vi "main.vi"() -> ()   [LabVIEW 2023] (continued)
00000004    8        68\t00\t97\tCC\t00\t16\t39\t8B\r\n      2262  1FFFFFFF   00000004    8        00\t00\tFF\tFF\tFF\tFF\tFF\tFF\r\n      2252  1FFFFFFF   00000004    8        00\t20\tFF\tFF\tFF\tFF\tFF\tFF\r\n      2247  1FFFFFFF   00000004    8        00\t00\tFF\tFF\tFF\tFF\tFF\tFF\r\n      2302  1FFFFFFF   00000004    8        00\t00\tFF\tFF\tFF\tFF\tFF\tFF\r\n      2293  18F106A7   00000004    8        00\tF7\tFF\tFF\tFF\tFF\tFF\t9E\r\n      2292  1FFFFFFF   00000004    8        00\t20\tFF\tFF\tFF\tFF\tFF\tFF\r\n      2283  0CF102A7   00000004    8        30\t75\tE0\t2E\t80\tFF\tFF\tFD\r\n      2283  0CF101A7   00000004    8        68\t00\t97\tCC\t00\t16\t39\t8C\r\n      2282  1FFFFFFF   00000004    8        00\t20\tFF\tFF\tFF\tFF\tFF\tFF\r\n      2272  1FFFFFFF   00000004    8        00\t20\tFF\tFF\tFF\tFF\tFF\tFF\r\n      2263  0CF102A7   00000004    8        30\t75\tE0\t2E\t80\tFF\tFF\tFD\r\n      2263  0CF101A7   00000004    8        68\t00\t97\tCC\t00\t16\t39\t8B\r\n      2262  1FFFFFFF   00000004    8        00\t00\tFF\tFF\tFF\tFF\tFF\tFF\r\n      2252  1FFFFFFF   00000004    8        00\t20\tFF\tFF\tFF\tFF\tFF\tFF\r\n      2303  0CF101A7   00000004    8        68\t00\t97\tCC\t00\t16\t39\t8D\r\n      2302  1FFFFFFF   00000004    8        00\t00\tFF\tFF\tFF\tFF\tFF\tFF\r\n      2293  18F106A7   00000004    8        00\tF7\tFF\tFF\tFF\tFF\tFF\t9E\r\n      2292  1FFFFFFF   00000004    8        00\t20\tFF\tFF\tFF\tFF\tFF\tFF\r\n      2283  0CF102A7   00000004    8        30\t75\tE0\t2E\t80\tFF\tFF\tFD\r\n      2283  0CF101A7   00000004    8        68\t00\t97\tCC\t00\t16\t39\t8C\r\n      2282  1FFFFFFF   00000004    8        00\t20\tFF\tFF\tFF\tFF\tFF\tFF\r\n      2272  1FFFFFFF   00000004    8        00\t20\tFF\tFF\tFF\tFF\tFF\tFF\r\n      2263  0CF102A7   00000004    8        30\t75\tE0\t2E\t80\tFF\tFF\tFD\r\n      2263  0CF101A7   00000004    8        68\t00\t97\tCC\t00\t16\t39\t8B\r\n      2262  1FFFFFFF   00000004    8        00\t00\tFF\tFF\tFF\tFF\tFF\tFF\r\n      2303  0CF102A7   00000004    8        30\t75\tE0\t2E\t80\tFF\tFF\tFD\r\n      2303  0CF101A7   00000004    8        68\t00\t97\tCC\t00\t16\t39\t8D\r\n      2302  1FFFFFFF   00000004    8        00\t00\tFF\tFF\tFF\tFF\tFF\tFF\r\n      2293  18F106A7   00000004    8        00\tF7\tFF\tFF\tFF\tFF\tFF\t9E\r\n      2292  1FFFFFFF   00000004    8        00\t20\tFF\tFF\tFF\tFF\tFF\tFF\r\n      2283  0CF102A7   00000004    8        30\t75\tE0\t2E\t80\tFF\tFF\tFD\r\n      2283  0CF101A7   00000004    8        68\t00\t97\tCC\t00\t16\t39\t8C\r\n      2282  1FFFFFFF   00000004    8        00\t20\tFF\tFF\tFF\tFF\tFF\tFF\r\n      2272  1FFFFFFF   00000004    8        00\t20\tFF\tFF\tFF\tFF\tFF\tFF\r\n      2263  0CF102A7   00000004    8        30\t75\tE0\t2E\t80\tFF\tFF\tFD\r\n      2263  0CF101A7   00000004    8        68\t00\t97\tCC\t00\t16\t39\t8B\r\n      2312  1FFFFFFF   00000004    8        00\t20\tFF\tFF\tFF\tFF\tFF\tFF\r\n      2303  0CF102A7   00000004    8        30\t75\tE0\t2E\t80\tFF\tFF\tFD\r\n      2303  0CF101A7   00000004    8        68\t00\t97\tCC\t00\t16\t39\t8D\r\n      2302  1FFFFFFF   00000004    8        00\t00\tFF\tFF\tFF\tFF\tFF\tFF\r\n      2293  18F106A7   00000004    8        00\tF7\tFF\tFF\tFF\tFF\tFF\t9E\r\n      2292  1FFFFFFF   00000004    8        00\t20\tFF\tFF\tFF\tFF\tFF\tFF\r\n      2283  0CF102A7   00000004    8        30\t75\tE0\t2E\t80\tFF\tFF\tFD\r\n      2283  0CF101A7   00000004    8        68\t00\t97\tCC\t00\t16\t39\t8C\r\n      2282  1FFFFFFF   00000004    8        00\t20\tFF\tFF\tFF\tFF\tFF\tFF\r\n      2272  1FFFFFFF   00000004    8        00\t20\tFF\tFF\tFF\tFF\tFF\tFF\r\n      2263  0CF102A7   00000004    8        30\t75\tE0\t2E\t80\tFF\tFF\tFD\r\n      2322  1FFFFFFF   00000004    8        00\t00\tFF\tFF\tFF\tFF\tFF\tFF\r\n      2312  1FFFFFFF   00000004    8        00\t20\tFF\tFF\tFF\tFF\tFF\tFF\r\n      2303  0CF102A7   00000004    8        30\t75\tE0\t2E\t80\tFF\tFF\tFD\r\n      2303  0CF101A7   00000004    8        68\t00\t97\tCC\t00\t16\t39\t8D\r\n      2302  1FFFFFFF   00000004    8        00\t00\tFF\tFF\tFF\tFF\tFF\tFF\r\n      2293  18F106A7   00000004    8        00\tF7\tFF\tFF\tFF\tFF\tFF\t9E\r\n      2292  1FFFFFFF   00000004    8        00\t20\tFF\tFF\tFF\tFF\tFF\tFF\r\n      2283  0CF102A7   00000004    8        30\t75\tE0\t2E\t80\tFF\tFF\tFD\r\n      2283  0CF101A7   00000004    8        68\t00\t97\tCC\t00\t16\t39\t8C\r\n      2282  1FFFFFFF   00000004    8        00\t20\tFF\tFF\tFF\tFF\tFF\tFF\r\n      2272  1FFFFFFF   00000004    8        00\t20\tFF\tFF\tFF\tFF\tFF\tFF\r\n      2323  0CF101A7   00000004    8        68\t00\t97\tCC\t00\t16\t39\t8E\r\n      2322  1FFFFFFF   00000004    8        00\t00\tFF\tFF\tFF\tFF\tFF\tFF\r\n      2312  1FFFFFFF   00000004    8        00\t20\tFF\tFF\tFF\tFF\tFF\tFF\r\n      2303  0CF102A7   00000004    8        30\t75\tE0\t2E\t80\tFF\tFF\tFD\r\n      2303  0CF101A7   00000004    8        68\t00\t97\tCC\t00\t16\t39\t8D\r\n      2302  1FFFFFFF   00000004    8        00\t00\tFF\tFF\tFF\tFF\tFF\tFF\r\n      2293  18F106A7   00000004    8        00\tF7\tFF\tFF\tFF\tFF\tFF\t9E\r\n      2292  1FFFFFFF   00000004    8        00\t20\tFF\tFF\tFF\tFF\tFF\tFF\r\n      2283  0CF102A7   00000004    8        30\t75\tE0\t2E\t80\tFF\tFF\tFD\r\n      2283  0CF101A7   00000004    8        68\t00\t97\tCC\t00\t16\t39\t8C\r\n      2282  1FFFFFFF   00000004    8        00\t20\tFF\tFF\tFF\tFF\tFF\tFF\r\n      2323  0CF102A7   00000004    8        30\t75\tE0\t2E\t80\tFF\tFF\tFD\r\n      2323  0CF101A7   00000004    8        68\t00\t97\tCC\t00\t16\t39\t8E\r\n      2322  1FFFFFFF   00000004    8        00\t00\tFF\tFF\tFF\tFF\tFF\tFF\r\n      2312  1FFFFFFF   00000004    8        00\t20\tFF\tFF\tFF\tFF\tFF\tFF\r\n      2303  0CF102A7   00000004    8        30\t75\tE0\t2E\t80\tFF\tFF\tFD\r\n      2303  0CF101A7   00000004    8        68\t00\t97\tCC\t00\t16\t39\t8D\r\n      2302  1FFFFFFF   00000004    8        00\t00\tFF\tFF\tFF\tFF\tFF\tFF\r\n      2293  18F106A7   00000004    8        00\tF7\tFF\tFF\tFF\tFF\tFF\t9E\r\n      2292  1FFFFFFF   00000004    8        00\t20\tFF\tFF\tFF\tFF\tFF\tFF\r\n      2283  0CF102A7   00000004    8        30\t75\tE0\t2E\t80\tFF\tFF\tFD\r\n      2283  0CF101A7   00000004    8        68\t00\t97\tCC\t00\t16\t39\t8C\r\n      2332  1FFFFFFF   00000004    8        00\t20\tFF\tFF\tFF\tFF\tFF\tFF\r\n      2323  0CF102A7   00000004    8        30\t75\tE0\t2E\t80\tFF\tFF\tFD\r\n      2323  0CF101A7   00000004    8        68\t00\t97\tCC\t00\t16\t39\t8E\r\n      2322  1FFFFFFF   00000004    8        00\t00\tFF\tFF\tFF\tFF\tFF\tFF\r\n      2312  1FFFFFFF   00000004    8        00\t20\tFF\tFF\tFF\tFF\tFF\tFF\r\n      2303  0CF102A7   00000004    8        30\t75\tE0\t2E\t80\tFF\tFF\tFD\r\n      2303  0CF101A7   00000004    8        68\t00\t97\tCC\t00\t16\t39\t8D\r\n      2302  1FFFFFFF   00000004    8        00\t00\tFF\tFF\tFF\tFF\tFF\tFF\r\n      2293  18F106A7   00000004    8        00\tF7\tFF\tFF\tFF\tFF\tFF\t9E\r\n      2292  1FFFFFFF   00000004    8        00\t20\tFF\tFF\tFF\tFF\tFF\tFF\r\n      2283  0CF102A7   00000004    8        30\t75\tE0\t2E\t80\tFF\tFF\tFD\r\n      2341  18F11FF0   00000004    8        FF\t3F\t90\t68\t88\t1B\t10\tFC\r\n      2332  1FFFFFFF   00000004    8        00\t20\tFF\tFF\tFF\tFF\tFF\tFF\r\n      2323  0CF102A7   00000004    8        30\t75\tE0\t2E\t80\tFF\tFF\tFD\r\n      2323  0CF101A7   00000004    8        68\t00\t97\tCC\t00\t16\t39\t8E\r\n      2322  1FFFFFFF   00000004    8        00\t00\tFF\tFF\tFF\tFF\tFF\tFF\r\n      2312  1FFFFFFF   00000004    8        00\t20\tFF\tFF\tFF\tFF\tFF\tFF\r\n      2303  0CF102A7   00000004    8        30\t75\tE0\t2E\t80\tFF\tFF\tFD\r\n      2303  0CF101A7   00000004    8        68\t00\t97\tCC\t00\t16\t39\t8D\r\n      2302  1FFFFFFF   00000004    8        00\t00\tFF\tFF\tFF\tFF\tFF\tFF\r\n      2293  18F106A7   00000004    8        00\tF7\tFF\tFF\tFF\tFF\tFF\t9E\r\n      2292  1FFFFFFF   00000004    8        00\t20\tFF\tFF\tFF\tFF\tFF\tFF\r\n      2342  18F120F0   00000004    8        2B\t75\t60\tB1\tB0\t01\tFF\tFF\r\n      2341  18F11FF0   00000004    8        FF\t3F\t90\t68\t88\t1B\t10\tFC\r\n      2332  1FFFFFFF   00000004    8        00\t20\tFF\tFF\tFF\tFF\tFF\tFF\r\n      2323  0CF102A7   00000004    8        30\t75\tE0\t2E\t80\tFF\tFF\tFD\r\n      2323  0CF101A7   00000004    8        68\t00\t97\tCC\t00\t16\t39\t8E\r\n      2322  1FFFFFFF   00000004    8        00\t00\tFF\tFF\tFF\tFF\tFF\tFF\r\n      2312  1FFFFFFF   00000004    8        00\t20\tFF\tFF\tFF\tFF\tFF\tFF\r\n      2303  0CF102A7   00000004    8        30\t75\tE0\t2E\t80\tFF\tFF\tFD\r\n      2303  0CF101A7   00000004    8        68\t00\t97\tCC\t00\t16\t39\t8D\r\n      2302  1FFFFFFF   00000004    8        00\t00\tFF\tFF\tFF\tFF\tFF\tFF\r\n      2293  18F106A7   00000004    8        00\tF7\tFF\tFF\tFF\tFF\tFF\t9E\r\n      2343  0CF101A7   00000004    8        68\t00\t97\tCC\t00\t16\t39\t8F\r\n      2342  18F120F0   00000004    8        2B\t75\t60\tB1\tB0\t01\tFF\tFF\r\n      2341  18F11FF0   00000004    8        FF\t3F\t90\t68\t88\t1B\t10\tFC\r\n      2332  1FFFFFFF   00000004    8        00\t20\tFF\tFF\tFF\tFF\tFF\tFF\r\n      2323  0CF102A7   00000004    8        30\t75\tE0\t2E\t80\tFF\tFF\tFD\r\n      2323  0CF101A7   00000004    8        68\t00\t97\tCC\t00\t16\t39\t8E\r\n      2322  1FFFFFFF   00000004    8        00\t00\tFF\tFF\tFF\tFF\tFF\tFF\r\n      2312  1FFFFFFF   00000004    8        00\t20\tFF\tFF\tFF\tFF\tFF\tFF\r\n      2303  0CF102A7   00000004    8        30\t75\tE0\t2E\t80\tFF\tFF\tFD\r\n      2303  0CF101A7   00000004    8        68\t00\t97\tCC\t00\t16\t39\t8D\r\n      2302  1FFFFFFF   00000004    8        00\t00\tFF\tFF\tFF\tFF\tFF\tFF\r\n      2343  0C3C4D4A   00000004    8        BE\tFF\tFF\t7F\t18\tFF\tFF\t4F\r\n      2343  0CF101A7   00000004    8        68\t00\t97\tCC\t00\t16\t39\t8F\r\n      2342  18F120F0   00000004    8        2B\t75\t60\tB1\tB0\t01\tFF\tFF\r\n      2341  18F11FF0   00000004    8        FF\t3F\t90\t68\t88\t1B\t10\tFC\r\n      2332  1FFFFFFF   00000004    8        00\t20\tFF\tFF\tFF\tFF\tFF\tFF\r\n      2323  0CF102A7   00000004    8        30\t75\tE0\t2E\t80\tFF\tFF\tFD\r\n      2323  0CF101A7   00000004    8        68\t00\t97\tCC\t00\t16\t39\t8E\r\n      2322  1FFFFFFF   00000004    8        00\t00\tFF\tFF\tFF\tFF\tFF\tFF\r\n      2312  1FFFFFFF   00000004    8        00\t20\tFF\tFF\tFF\tFF\tFF\tFF\r\n      2303  0CF102A7   00000004    8        30\t75\tE0\t2E\t80\tFF\tFF\tFD\r\n      2303  0CF101A7   00000004    8        68\t00\t97\tCC\t00\t16\t39\t8D\r\n      2344  0CF102A7   00000004    8        30\t75\tE0\t2E\t80\tFF\tFF\tFD\r\n      2343  0C3C4D4A   00000004    8        BE\tFF\tFF\t7F\t18\tFF\tFF\t4F\r\n      2343  0CF101A7   00000004    8        68\t00\t97\tCC\t00\t16\t39\t8F\r\n      2342  18F120F0   00000004    8        2B\t75\t60\tB1\tB0\t01\tFF\tFF\r\n      2341  18F11FF0   00000004    8        FF\t3F\t90\t68\t88\t1B\t10\tFC\r\n      2332  1FFFFFFF   00000004    8        00\t20\tFF\tFF\tFF\tFF\tFF\tFF\r\n      2323  0CF102A7   00000004    8        30\t75\tE0\t2E\t80\tFF\tFF\tFD\r\n      2323  0CF101A7   00000004    8        68\t00\t97\tCC\t00\t16\t39\t8E\r\n      2322  1FFFFFFF   00000004    8        00\t00\tFF\tFF\tFF\tFF\tFF\tFF\r\n      2312  1FFFFFFF   00000004    8        00\t20\tFF\tFF\tFF\tFF\tFF\tFF\r\n      2303  0CF102A7   00000004    8        30\t75\tE0\t2E\t80\tFF\tFF\tFD\r\n      2344  0CF103A7   00000004    8        17\t1F\t08\t60\tB1\t1F\t08\t4F\r\n      2344  0CF102A7   00000004    8        30\t75\tE0\t2E\t80\tFF\tFF\tFD\r\n      2343  0C3C4D4A   00000004    8        BE\tFF\tFF\t7F\t18\tFF\tFF\t4F\r\n      2343  0CF101A7   00000004    8        68\t00\t97\tCC\t00\t16\t39\t8F\r\n      2342  18F120F0   00000004    8        2B\t75\t60\tB1\tB0\t01\tFF\tFF\r\n      2341  18F11FF0   00000004    8        FF\t3F\t90\t68\t88\t1B\t10\tFC\r\n      2332  1FFFFFFF   00000004    8        00\t20\tFF\tFF\tFF\tFF\tFF\tFF\r\n      2323  0CF102A7   00000004    8        30\t75\tE0\t2E\t80\tFF\tFF\tFD\r\n      2323  0CF101A7   00000004    8        68\t00\t97\tCC\t00\t16\t39\t8E\r\n      2322  1FFFFFFF   00000004    8        00\t00\tFF\tFF\tFF\tFF\tFF\tFF\r\n      2312  1FFFFFFF   00000004    8        00\t20\tFF\tFF\tFF\tFF\tFF\tFF\r\n      2345  0CF104A7   00000004    8        F0\t60\t22\tFC\tFF\tFF\tFF\t4F\r\n      2344  0CF103A7   00000004    8        17\t1F\t08\t60\tB1\t1F\t08\t4F\r\n      2344  0CF102A7   00000004    8        30\t75\tE0\t2E\t80\tFF\tFF\tFD\r\n      2343  0C3C4D4A   00000004    8        BE\tFF\tFF\t7F\t18\tFF\tFF\t4F\r\n      2343  0CF101A7   00000004    8        68\t00\t97\tCC\t00\t16\t39\t8F\r\n      2342  18F120F0   00000004    8        2B\t75\t60\tB1\tB0\t01\tFF\tFF\r\n      2341  18F11FF0   00000004    8        FF\t3F\t90\t68\t88\t1B\t10\tFC\r\n      2332  1FFFFFFF   00000004    8        00\t20\tFF\tFF\tFF\tFF\tFF\tFF\r\n      2323  0CF102A7   00000004    8        30\t75\tE0\t2E\t80\tFF\tFF\tFD\r\n      2323  0CF101A7   00000004    8        68\t00\t97\tCC\t00\t16\t39\t8E\r\n      2322  1FFFFFFF   00000004    8        00\t00\tFF\tFF\tFF\tFF\tFF\tFF\r\n      2345  18F106A7   00000004    8        00\tF7\tFF\tFF\tFF\tFF\tFF\t9F\r\n      2345  0CF104A7   00000004    8        F0\t60\t22\tFC\tFF\tFF\tFF\t4F\r\n      2344  0CF103A7   00000004    8        17\t1F\t08\t60\tB1\t1F\t08\t4F\r\n      2344  0CF102A7   00000004    8        30\t75\tE0\t2E\t80\tFF\tFF\tFD\r\n      2343  0C3C4D4A   00000004    8        BE\tFF\tFF\t7F\t18\tFF\tFF\t4F\r\n      2343  0CF101A7   00000004    8        68\t00\t97\tCC\t00\t16\t39\t8F\r\n      2342  18F120F0   00000004    8        2B\t75\t60\tB1\tB0\t01\tFF\tFF\r\n      2341  18F11FF0   00000004    8        FF\t3F\t90\t68\t88\t1B\t10\tFC\r\n      2332  1FFFFFFF   00000004    8        00\t20\tFF\tFF\tFF\tFF\tFF\tFF\r\n      2323  0CF102A7   00000004    8        30\t75\tE0\t2E\t80\tFF\tFF\tFD\r\n      2323  0CF101A7   00000004    8        68\t00\t97\tCC\t00\t16\t39\t8E\r\n      2346  18F121F0   00000004    8        09\t19\t00\t00\tFF\tFF\tB0\t01\r\n      2345  18F106A7   00000004    8        00\tF7\tFF\tFF\tFF\tFF\tFF\t9F\r\n      2345  0CF104A7   00000004    8        F0\t60\t22\tFC\tFF\tFF\tFF\t4F\r\n      2344  0CF103A7   00000004    8        17\t1F\t08\t60\tB1\t1F\t08\t4F\r\n      2344  0CF102A7   00000004    8        30\t75\tE0\t2E\t80\tFF\tFF\tFD\r\n      2343  0C3C4D4A   00000004    8        BE\tFF\tFF\t7F\t18\tFF\tFF\t4F\r\n      2343  0CF101A7   00000004    8        68\t00\t97\tCC\t00\t16\t39\t8F\r\n      2342  18F120F0   00000004    8        2B\t75\t60\tB1\tB0\t01\tFF\tFF\r\n      2341  18F11FF0   00000004    8        FF\t3F\t90\t68\t88\t1B\t10\tFC\r\n      2332  1FFFFFFF   00000004    8        00\t20\tFF\tFF\tFF\tFF\tFF\tFF\r\n      2323  0CF102A7   00000004    8        30\t75\tE0\t2E\t80\tFF\tFF\tFD\r\n      2347  1FFFFFFF   00000004    8        00\t20\tFF\tFF\tFF\tFF\tFF\tFF\r\n      2346  18F121F0   00000004    8        09\t19\t00\t00\tFF\tFF\tB0\t01\r\n      2345  18F106A7   00000004    8        00\tF7\tFF\tFF\tFF\tFF\tFF\t9F\r\n      2345  0CF104A7   00000004    8        F0\t60\t22\tFC\tFF\tFF\tFF\t4F\r\n      2344  0CF103A7   00000004    8        17\t1F\t08\t60\tB1\t1F\t08\t4F\r\n      2344  0CF102A7   00000004    8        30\t75\tE0\t2E\t80\tFF\tFF\tFD\r\n      2343  0C3C4D4A   00000004    8        BE\tFF\tFF\t7F\t18\tFF\tFF\t4F\r\n      2343  0CF101A7   00000004    8        68\t00\t97\tCC\t00\t16\t39\t8F\r\n      2342  18F120F0   00000004    8        2B\t75\t60\tB1\tB0\t01\tFF\tFF\r\n      2341  18F11FF0   00000004    8        FF\t3F\t90\t68\t88\t1B\t10\tFC\r\n      2332  1FFFFFFF   00000004    8        00\t20\tFF\tFF\tFF\tFF\tFF\tFF\r\n      2352  1FFFFFFF   00000004    8        00\t20\tFF\tFF\tFF\tFF\tFF\tFF\r\n      2347  1FFFFFFF   00000004    8        00\t20\tFF\tFF\tFF\tFF\tFF\tFF\r\n      2346  18F121F0   00000004    8        09\t19\t00\t00\tFF\tFF\tB0\t01\r\n      2345  18F106A7   00000004    8        00\tF7\tFF\tFF\tFF\tFF\tFF\t9F\r\n      2345  0CF104A7   00000004    8        F0\t60\t22\tFC\tFF\tFF\tFF\t4F\r\n      2344  0CF103A7   00000004    8        17\t1F\t08\t60\tB1\t1F\t08\t4F\r\n      2344  0CF102A7   00000004    8        30\t75\tE0\t2E\t80\tFF\tFF\tFD\r\n      2343  0C3C4D4A   00000004    8        BE\tFF\tFF\t7F\t18\tFF\tFF\t4F\r\n      2343  0CF101A7   00000004    8        68\t00\t97\tCC\t00\t16\t39\t8F\r\n      2342  18F120F0   00000004    8        2B\t75\t60\tB1\tB0\t01\tFF\tFF\r\n      2341  18F11FF0   00000004    8        FF\t3F\t90\t68\t88\t1B\t10\tFC\r\n      2362  1FFFFFFF   00000004    8        00\t00\tFF\tFF\tFF\tFF\tFF\tFF\r\n      2352  1FFFFFFF   00000004    8        00\t20\tFF\tFF\tFF\tFF\tFF\tFF\r\n      2347  1FFFFFFF   00000004    8        00\t20\tFF\tFF\tFF\tFF\tFF\tFF\r\n      2346  18F121F0   00000004    8        09\t19\t00\t00\tFF\tFF\tB0\t01\r\n      2345  18F106A7   00000004    8        00\tF7\tFF\tFF\tFF\tFF\tFF\t9F\r\n      2345  0CF104A7   00000004    8        F0\t60\t22\tFC\tFF\tFF\tFF\t4F\r\n      2344  0CF103A7   00000004    8        17\t1F\t08\t60\tB1\t1F\t08\t4F\r\n      2344  0CF102A7   00000004    8        30\t75\tE0\t2E\t80\tFF\tFF\tFD\r\n      2343  0C3C4D4A   00000004    8        BE\tFF\tFF\t7F\t18\tFF\tFF\t4F\r\n      2343  0CF101A7   00000004    8        68\t00\t97\tCC\t00\t16\t39\t8F\r\n      2342  18F120F0   00000004    8        2B\t75\t60\tB1\tB0\t01\tFF\tFF\r\n      2363  0CF101A7   00000004    8        68\t00\t97\tCC\t00\t16\t39\t90\r\n      2362  1FFFFFFF   00000004    8        00\t00\tFF\tFF\tFF\tFF\tFF\tFF\r\n      2352  1FFFFFFF   00000004    8        00\t20\tFF\tFF\tFF\tFF\tFF\tFF\r\n      2347  1FFFFFFF   00000004    8        00\t20\tFF\tFF\tFF\tFF\tFF\tFF\r\n      2346  18F121F0   00000004    8        09\t19\t00\t00\tFF\tFF\tB0\t01\r\n      2345  18F106A7   00000004    8        00\tF7\tFF\tFF\tFF\tFF\tFF\t9F\r\n      2345  0CF104A7   00000004    8        F0\t60\t22\tFC\tFF\tFF\tFF\t4F\r\n      2344  0CF103A7   00000004    8        17\t1F\t08\t60\tB1\t1F\t08\t4F\r\n      2344  0CF102A7   00000004    8        30\t75\tE0\t2E\t80\tFF\tFF\tFD\r\n      2343  0C3C4D4A   00000004    8        BE\tFF\tFF\t7F\t18\tFF\tFF\t4F\r\n      2343  0CF101A7   00000004    8        68\t00\t97\tCC\t00\t16\t39\t8F\r\n      2363  0CF102A7   00000004    8        30\t75\tE0\t2E\t80\tFF\tFF\tFD\r\n      2363  0CF101A7   00000004    8        68\t00\t97\tCC\t00\t16\t39\t90\r\n      2362  1FFFFFFF   00000004    8        00\t00\tFF\tFF\tFF\tFF\tFF\tFF\r\n      2352  1FFFFFFF   00000004    8        00\t20\tFF\tFF\tFF\tFF\tFF\tFF\r\n      2347  1FFFFFFF   00000004    8        00\t20\tFF\tFF\tFF\tFF\tFF\tFF\r\n      2346  18F121F0   00000004    8        09\t19\t00\t00\tFF\tFF\tB0\t01\r\n      2345  18F106A7   00000004    8        00\tF7\tFF\tFF\tFF\tFF\tFF\t9F\r\n      2345  0CF104A7   00000004    8        F0\t60\t22\tFC\tFF\tFF\tFF\t4F\r\n      2344  0CF103A7   00000004    8        17\t1F\t08\t60\tB1\t1F\t08\t4F\r\n      2344  0CF102A7   00000004    8        30\t75\tE0\t2E\t80\tFF\tFF\tFD\r\n      2343  0C3C4D4A   00000004    8        BE\tFF\tFF\t7F\t18\tFF\tFF\t4F\r\n      2372  1FFFFFFF   00000004    8        00\t20\tFF\tFF\tFF\tFF\tFF\tFF\r\n      2363  0CF102A7   00000004    8        30\t75\tE0\t2E\t80\tFF\tFF\tFD\r\n      2363  0CF101A7   00000004    8        68\t00\t97\tCC\t00\t16\t39\t90\r\n      2362  1FFFFFFF   00000004    8        00\t00\tFF\tFF\tFF\tFF\tFF\tFF\r\n      2352  1FFFFFFF   00000004    8        00\t20\tFF\tFF\tFF\tFF\tFF\tFF\r\n      2347  1FFFFFFF   00000004    8        00\t20\tFF\tFF\tFF\tFF\tFF\tFF\r\n      2346  18F121F0   00000004    8        09\t19\t00\t00\tFF\tFF\tB0\t01\r\n      2345  18F106A7   00000004    8        00\tF7\tFF\tFF\tFF\tFF\tFF\t9F\r\n      2345  0CF104A7   00000004    8        F0\t60\t22\tFC\tFF\tFF\tFF\t4F\r\n      2344  0CF103A7   00000004    8        17\t1F\t08\t60\tB1\t1F\t08\t4F\r\n      2344  0CF102A7   00000004    8        30\t75\tE0\t2E\t80\tFF\tFF\tFD\r\n      2382  1FFFFFFF   00000004    8        00\t20\tFF\tFF\tFF\tFF\tFF\tFF\r\n      2372  1FFFFFFF   00000004    8        00\t20\tFF\tFF\tFF\tFF\tFF\tFF\r\n      2363  0CF102A7   00000004    8        30\t75\tE0\t2E\t80\tFF\tFF\tFD\r\n      2363  0CF101A7   00000004    8        68\t00\t97\tCC\t00\t16\t39\t90\r\n      2362  1FFFFFFF   00000004    8        00\t00\tFF\tFF\tFF\tFF\tFF\tFF\r\n      2352  1FFFFFFF   00000004    8        00\t20\tFF\tFF\tFF\tFF\tFF\tFF\r\n      2347  1FFFFFFF   00000004    8        00\t20\tFF\tFF\tFF\tFF\tFF\tFF\r\n      2346  18F121F0   00000004    8        09\t19\t00\t00\tFF\tFF\tB0\t01\r\n      2345  18F106A7   00000004    8        00\tF7\tFF\tFF\tFF\tFF\tFF\t9F\r\n      2345  0CF104A7   00000004    8        F0\t60\t22\tFC\tFF\tFF\tFF\t4F\r\n      2344  0CF103A7   00000004    8        17\t1F\t08\t60\tB1\t1F\t08\t4F\r\n      2383  0CF101A7   00000004    8        68\t00\t97\tCC\t00\t16\t39\t91\r\n      2382  1FFFFFFF   00000004    8        00\t20\tFF\tFF\tFF\tFF\tFF\tFF\r\n      2372  1FFFFFFF   00000004    8        00\t20\tFF\tFF\tFF\tFF\tFF\tFF\r\n      2363  0CF102A7   00000004    8        30\t75\tE0\t2E\t80\tFF\tFF\tFD\r\n      2363  0CF101A7   00000004    8        68\t00\t97\tCC\t00\t16\t39\t90\r\n      2362  1FFFFFFF   00000004    8        00\t00\tFF\tFF\tFF\tFF\tFF\tFF\r\n      2352  1FFFFFFF   00000004    8        00\t20\tFF\tFF\tFF\tFF\tFF\tFF\r\n      2347  1FFFFFFF   00000004    8        00\t20\tFF\tFF\tFF\tFF\tFF\tFF\r\n      2346  18F121F0   00000004    8        09\t19\t00\t00\tFF\tFF\tB0\t01\r\n      2345  18F106A7   00000004    8        00\tF7\tFF\tFF\tFF\tFF\tFF\t9F\r\n      2345  0CF104A7   00000004    8        F0\t60\t22\tFC\tFF\tFF\tFF\t4F\r\n      2383  0CF102A7   00000004    8        30\t75\tE0\t2E\t80\tFF\tFF\tFD\r\n      2383  0CF101A7   00000004    8        68\t00\t97\tCC\t00\t16\t39\t91\r\n      2382  1FFFFFFF   00000004    8        00\t20\tFF\tFF\tFF\tFF\tFF\tFF\r\n      2372  1FFFFFFF   00000004    8        00\t20\tFF\tFF\tFF\tFF\tFF\tFF\r\n      2363  0CF102A7   00000004    8        30\t75\tE0\t2E\t80\tFF\tFF\tFD\r\n      2363  0CF101A7   00000004    8        68\t00\t97\tCC\t00\t16\t39\t90\r\n      2362  1FFFFFFF   00000004    8        00\t00\tFF\tFF\tFF\tFF\tFF\tFF\r\n      2352  1FFFFFFF   00000004    8        00\t20\tFF\tFF\tFF\tFF\tFF\tFF\r\n      2347  1FFFFFFF   00000004    8        00\t20\tFF\tFF\tFF\tFF\tFF\tFF\r\n      2346  18F121F0   00000004    8        09\t19\t00\t00\tFF\tFF\tB0\t01\r\n      2345  18F106A7   00000004    8        00\tF7\tFF\tFF\tFF\tFF\tFF\t9F\r\n      2392  1FFFFFFF   00000004    8        00\t20\tFF\tFF\tFF\tFF\tFF\tFF\r\n      2383  0CF102A7   00000004    8        30\t75\tE0\t2E\t80\tFF\tFF\tFD\r\n      2383  0CF101A7   00000004    8        68\t00\t97\tCC\t00\t16\t39\t91\r\n      2382  1FFFFFFF   00000004    8        00\t20\tFF\tFF\tFF\tFF\tFF\tFF\r\n      2372  1FFFFFFF   00000004    8        00\t20\tFF\tFF\tFF\tFF\tFF\tFF\r\n      2363  0CF102A7   00000004    8        30\t75\tE0\t2E\t80\tFF\tFF\tFD\r\n      2363  0CF101A7   00000004    8        68\t00\t97\tCC\t00\t16\t39\t90\r\n      2362  1FFFFFFF   00000004    8        00\t00\tFF\tFF\tFF\tFF\tFF\tFF\r\n      2352  1FFFFFFF   00000004    8        00\t20\tFF\tFF\tFF\tFF\tFF\tFF\r\n      2347  1FFFFFFF   00000004    8        00\t20\tFF\tFF\tFF\tFF\tFF\tFF\r\n      2346  18F121F0   00000004    8        09\t19\t00\t00\tFF\tFF\tB0\t01\r\n      2393  18F106A7   00000004    8        00\tF7\tFF\tFF\tFF\tFF\tFF\tA0\r\n      2392  1FFFFFFF   00000004    8        00\t20\tFF\tFF\tFF\tFF\tFF\tFF\r\n      2383  0CF102A7   00000004    8        30\t75\tE0\t2E\t80\tFF\tFF\tFD\r\n      2383  0CF101A7   00000004    8        68\t00\t97\tCC\t00\t16\t39\t91\r\n      2382  1FFFFFFF   00000004    8        00\t20\tFF\tFF\tFF\tFF\tFF\tFF\r\n      2372  1FFFFFFF   00000004    8        00\t20\tFF\tFF\tFF\tFF\tFF\tFF\r\n      2363  0CF102A7   00000004    8        30\t75\tE0\t2E\t80\tFF\tFF\tFD\r\n      2363  0CF101A7   00000004    8        68\t00\t97\tCC\t00\t16\t39\t90\r\n      2362  1FFFFFFF   00000004    8        00\t00\tFF\tFF\tFF\tFF\tFF\tFF\r\n      2352  1FFFFFFF   00000004    8        00\t20\tFF\tFF\tFF\tFF\tFF\tFF\r\n      2347  1FFFFFFF   00000004    8        00\t20\tFF\tFF\tFF\tFF\tFF\tFF\r\n      2402  1FFFFFFF   00000004    8        00\t00\tFF\tFF\tFF\tFF\tFF\tFF\r\n      2393  18F106A7   00000004    8        00\tF7\tFF\tFF\tFF\tFF\tFF\tA0\r\n      2392  1FFFFFFF   00000004    8        00\t20\tFF\tFF\tFF\tFF\tFF\tFF\r\n      2383  0CF102A7   00000004    8        30\t75\tE0\t2E\t80\tFF\tFF\tFD\r\n      2383  0CF101A7   00000004    8        68\t00\t97\tCC\t00\t16\t39\t91\r\n      2382  1FFFFFFF   00000004    8        00\t20\tFF\tFF\tFF\tFF\tFF\tFF\r\n      2372  1FFFFFFF   00000004    8        00\t20\tFF\tFF\tFF\tFF\tFF\tFF\r\n      2363  0CF102A7   00000004    8        30\t75\tE0\t2E\t80\tFF\tFF\tFD\r\n      2363  0CF101A7   00000004    8        68\t00\t97\tCC\t00\t16\t39\t90\r\n      2362  1FFFFFFF   00000004    8        00\t00\tFF\tFF\tFF\tFF\tFF\tFF\r\n      2352  1FFFFFFF   00000004    8        00\t20\tFF\tFF\tFF\tFF\tFF\tFF\r\n      2403  0CF101A7   00000004    8        68\t00\t97\tCC\t00\t16\t39\t92\r\n      2402  1FFFFFFF   00000004    8        00\t00\tFF\tFF\tFF\tFF\tFF\tFF\r\n      2393  18F106A7   00000004    8        00\tF7\tFF\tFF\tFF\tFF\tFF\tA0\r\n      2392  1FFFFFFF   00000004    8        00\t20\tFF\tFF\tFF\tFF\tFF\tFF\r\n      2383  0CF102A7   00000004    8        30\t75\tE0\t2E\t80\tFF\tFF\tFD\r\n      2383  0CF101A7   00000004    8        68\t00\t97\tCC\t00\t16\t39\t91\r\n      2382  1FFFFFFF   00000004    8        00\t20\tFF\tFF\tFF\tFF\tFF\tFF\r\n      2372  1FFFFFFF   00000004    8        00\t20\tFF\tFF\tFF\tFF\tFF\tFF\r\n      2363  0CF102A7   00000004    8        30\t75\tE0\t2E\t80\tFF\tFF\tFD\r\n      2363  0CF101A7   00000004    8        68\t00\t97\tCC\t00\t16\t39\t90\r\n      2362  1FFFFFFF   00000004    8        00\t00\tFF\tFF\tFF\tFF\tFF\tFF\r\n      2403  0CF102A7   00000004    8        30\t75\tE0\t2E\t80\tFF\tFF\tFD\r\n      2403  0CF101A7   00000004    8        68\t00\t97\tCC\t00\t16\t39\t92\r\n      2402  1FFFFFFF   00000004    8        00\t00\tFF\tFF\tFF\tFF\tFF\tFF\r\n      2393  18F106A7   00000004    8        00\tF7\tFF\tFF\tFF\tFF\tFF\tA0\r\n      2392  1FFFFFFF   00000004    8        00\t20\tFF\tFF\tFF\tFF\tFF\tFF\r\n      2383  0CF102A7   00000004    8        30\t75\tE0\t2E\t80\tFF\tFF\tFD\r\n      2383  0CF101A7   00000004    8        68\t00\t97\tCC\t00\t16\t39\t91\r\n      2382  1FFFFFFF   00000004    8        00\t20\tFF\tFF\tFF\tFF\tFF\tFF\r\n      2372  1FFFFFFF   00000004    8        00\t20\tFF\tFF\tFF\tFF\tFF\tFF\r\n      2363  0CF102A7   00000004    8        30\t75\tE0\t2E\t80\tFF\tFF\tFD\r\n      2363  0CF101A7   00000004    8        68\t00\t97\tCC\t00\t16\t39\t90\r\n      2412  1FFFFFFF   00000004    8        00\t20\tFF\tFF\tFF\tFF\tFF\tFF\r\n      2403  0CF102A7   00000004    8        30\t75\tE0\t2E\t80\tFF\tFF\tFD\r\n      2403  0CF101A7   00000004    8        68\t00\t97\tCC\t00\t16\t39\t92\r\n      2402  1FFFFFFF   00000004    8        00\t00\tFF\tFF\tFF\tFF\tFF\tFF\r\n      2393  18F106A7   00000004    8        00\tF7\tFF\tFF\tFF\tFF\tFF\tA0\r\n      2392  1FFFFFFF   00000004    8        00\t20\tFF\tFF\tFF\tFF\tFF\tFF\r\n      2383  0CF102A7   00000004    8        30\t75\tE0\t2E\t80\tFF\tFF\tFD\r\n      2383  0CF101A7   00000004    8        68\t00\t97\tCC\t00\t16\t39\t91\r\n      2382  1FFFFFFF   00000004    8        00\t20\tFF\tFF\tFF\tFF\tFF\tFF\r\n      2372  1FFFFFFF   00000004    8        00\t20\tFF\tFF\tFF\tFF\tFF\tFF\r\n      2363  0CF102A7   00000004    8        30\t75\tE0\t2E\t80\tFF\tFF\tFD\r\n      2422  1FFFFFFF   00000004    8        00\t00\tFF\tFF\tFF\tFF\tFF\tFF\r\n      2412  1FFFFFFF   00000004    8        00\t20\tFF\tFF\tFF\tFF\tFF\tFF\r\n      2403  0CF102A7   00000004    8        30\t75\tE0\t2E\t80\tFF\tFF\tFD\r\n      2403  0CF101A7   00000004    8        68\t00\t97\tCC\t00\t16\t39\t92\r\n      2402  1FFFFFFF   00000004    8        00\t00\tFF\tFF\tFF\tFF\tFF\tFF\r\n      2393  18F106A7   00000004    8        00\tF7\tFF\tFF\tFF\tFF\tFF\tA0\r\n      2392  1FFFFFFF   00000004    8        00\t20\tFF\tFF\tFF\tFF\tFF\tFF\r\n      2383  0CF102A7   00000004    8        30\t75\tE0\t2E\t80\tFF\tFF\tFD\r\n      2383  0CF101A7   00000004    8        68\t00\t97\tCC\t00\t16\t39\t91\r\n      2382  1FFFFFFF   00000004    8        00\t20\tFF\tFF\tFF\tFF\tFF\tFF\r\n      2372  1FFFFFFF   00000004    8        00\t20\tFF\tFF\tFF\tFF\tFF\tFF\r\n      2423  0CF101A7   00000004    8        68\t00\t97\tCC\t00\t16\t39\t93\r\n      2422  1FFFFFFF   00000004    8        00\t00\tFF\tFF\tFF\tFF\tFF\tFF\r\n      2412  1FFFFFFF   00000004    8        00\t20\tFF\tFF\tFF\tFF\tFF\tFF\r\n      2403  0CF102A7   00000004    8        30\t75\tE0\t2E\t80\tFF\tFF\tFD\r\n      2403  0CF101A7   00000004    8        68\t00\t97\tCC\t00\t16\t39\t92\r\n      2402  1FFFFFFF   00000004    8        00\t00\tFF\tFF\tFF\tFF\tFF\tFF\r\n      2393  18F106A7   00000004    8        00\tF7\tFF\tFF\tFF\tFF\tFF\tA0\r\n      2392  1FFFFFFF   00000004    8        00\t20\tFF\tFF\tFF\tFF\tFF\tFF\r\n      2383  0CF102A7   00000004    8        30\t75\tE0\t2E\t80\tFF\tFF\tFD\r\n      2383  0CF101A7   00000004    8        68\t00\t97\tCC\t00\t16\t39\t91\r\n      2382  1FFFFFFF   00000004    8        00\t20\tFF\tFF\tFF\tFF\tFF\tFF\r\n      2423  0CF102A7   00000004    8        30\t75\tE0\t2E\t80\tFF\tFF\tFD\r\n      2423  0CF101A7   00000004    8        68\t00\t97\tCC\t00\t16\t39\t93\r\n      2422  1FFFFFFF   00000004    8        00\t00\tFF\tFF\tFF\tFF\tFF\tFF\r\n      2412  1FFFFFFF   00000004    8        00\t20\tFF\tFF\tFF\tFF\tFF\tFF\r\n      2403  0CF102A7   00000004    8        30\t75\tE0\t2E\t80\tFF\tFF\tFD\r\n      2403  0CF101A7   00000004    8        68\t00\t97\tCC\t00\t16\t39\t92\r\n      2402  1FFFFFFF   00000004    8        00\t00\tFF\tFF\tFF\tFF\tFF\tFF\r\n      2393  18F106A7   00000004    8        00\tF7\tFF\tFF\tFF\tFF\tFF\tA0\r\n      2392  1FFFFFFF   00000004    8        00\t20\tFF\tFF\tFF\tFF\tFF\tFF\r\n      2383  0CF102A7   00000004    8        30\t75\tE0\t2E\t80\tFF\tFF\tFD\r\n      2383  0CF101A7   00000004    8        68\t00\t97\tCC\t00\t16\t39\t91\r\n      2432  1FFFFFFF   00000004    8        00\t20\tFF\tFF\tFF\tFF\tFF\tFF\r\n      2423  0CF102A7   00000004    8        30\t75\tE0\t2E\t80\tFF\tFF\tFD\r\n      2423  0CF101A7   00000004    8        68\t00\t97\tCC\t00\t16\t39\t93\r\n      2422  1FFFFFFF   00000004    8        00\t00\tFF\tFF\tFF\tFF\tFF\tFF\r\n      2412  1FFFFFFF   00000004    8        00\t20\tFF\tFF\tFF\tFF\tFF\tFF\r\n      2403  0CF102A7   00000004    8        30\t75\tE0\t2E\t80\tFF\tFF\tFD\r\n      2403  0CF101A7   00000004    8        68\t00\t97\tCC\t00\t16\t39\t92\r\n      2402  1FFFFFFF   00000004    8        00\t00\tFF\tFF\tFF\tFF\tFF\tFF\r\n      2393  18F106A7   00000004    8        00\tF7\tFF\tFF\tFF\tFF\tFF\tA0\r\n      2392  1FFFFFFF   00000004    8        00\t20\tFF\tFF\tFF\tFF\tFF\tFF\r\n      2383  0CF102A7   00000004    8        30\t75\tE0\t2E\t80\tFF\tFF\tFD\r\n      2441  18F11FF0   00000004    8        FF\t3F\t90\t68\t88\t1B\t10\t0C\r\n      2432  1FFFFFFF   00000004    8        00\t20\tFF\tFF\tFF\tFF\tFF\tFF\r\n      2423  0CF102A7   00000004    8        30\t75\tE0\t2E\t80\tFF\tFF\tFD\r\n      2423  0CF101A7   00000004    8        68\t00\t97\tCC\t00\t16\t39\t93\r\n      2422  1FFFFFFF   00000004    8        00\t00\tFF\tFF\tFF\tFF\tFF\tFF\r\n      2412  1FFFFFFF   00000004    8        00\t20\tFF\tFF\tFF\tFF\tFF\tFF\r\n      2403  0CF102A7   00000004    8        30\t75\tE0\t2E\t80\tFF\tFF\tFD\r\n      2403  0CF101A7   00000004    8        68\t00\t97\tCC\t00\t16\t39\t92\r\n      2402  1FFFFFFF   00000004    8        00\t00\tFF\tFF\tFF\tFF\tFF\tFF\r\n      2393  18F106A7   00000004    8        00\tF7\tFF\tFF\tFF\tFF\tFF\tA0\r\n      2392  1FFFFFFF   00000004    8        00\t20\tFF\tFF\tFF\tFF\tFF\tFF\r\n      2442  18F120F0   00000004    8        2B\t75\t60\tB1\tB0\t01\tFF\tFF\r\n      2441  18F11FF0   00000004    8        FF\t3F\t90\t68\t88\t1B\t10\t0C\r\n      2432  1FFFFFFF   00000004    8        00\t20\tFF\tFF\tFF\tFF\tFF\tFF\r\n      2423  0CF102A7   00000004    8        30\t75\tE0\t2E\t80\tFF\tFF\tFD\r\n      2423  0CF101A7   00000004    8        68\t00\t97\tCC\t00\t16\t39\t93\r\n      2422  1FFFFFFF   00000004    8        00\t00\tFF\tFF\tFF\tFF\tFF\tFF\r\n      2412  1FFFFFFF   00000004    8        00\t20\tFF\tFF\tFF\tFF\tFF\tFF\r\n      2403  0CF102A7   00000004    8        30\t75\tE0\t2E\t80\tFF\tFF\tFD\r\n      2403  0CF101A7   00000004    8        68\t00\t97\tCC\t00\t16\t39\t92\r\n      2402  1FFFFFFF   00000004    8        00\t00\tFF\tFF\tFF\tFF\tFF\tFF\r\n      2393  18F106A7   00000004    8        00\tF7\tFF\tFF\tFF\tFF\tFF\tA0\r\n      2443  0CF101A7   00000004    8        68\t00\t97\tCC\t00\t16\t39\t94\r\n      2442  18F120F0   00000004    8        2B\t75\t60\tB1\tB0\t01\tFF\tFF\r\n      2441  18F11FF0   00000004    8        FF\t3F\t90\t68\t88\t1B\t10\t0C\r\n      2432  1FFFFFFF   00000004    8        00\t20\tFF\tFF\tFF\tFF\tFF\tFF\r\n      2423  0CF102A7   00000004    8        30\t75\tE0\t2E\t80\tFF\tFF\tFD\r\n      2423  0CF101A7   00000004    8        68\t00\t97\tCC\t00\t16\t39\t93\r\n      2422  1FFFFFFF   00000004    8        00\t00\tFF\tFF\tFF\tFF\tFF\tFF\r\n      2412  1FFFFFFF   00000004    8        00\t20\tFF\tFF\tFF\tFF\tFF\tFF\r\n      2403  0CF102A7   00000004    8        30\t75\tE0\t2E\t80\tFF\tFF\tFD\r\n      2403  0CF101A7   00000004    8        68\t00\t97\tCC\t00\t16\t39\t92\r\n      2402  1FFFFFFF   00000004    8        00\t00\tFF\tFF\tFF\tFF\tFF\tFF\r\n      2443  0C3C4D4A   00000004    8        BE\tFF\tFF\t7F\t18\tFF\tFF\t50\r\n      2443  0CF101A7   00000004    8        68\t00\t97\tCC\t00\t16\t39\t94\r\n      2442  18F120F0   00000004    8        2B\t75\t60\tB1\tB0\t01\tFF\tFF\r\n      2441  18F11FF0   00000004    8        FF\t3F\t90\t68\t88\t1B\t10\t0C\r\n      2432  1FFFFFFF   00000004    8        00\t20\tFF\tFF\tFF\tFF\tFF\tFF\r\n      2423  0CF102A7   00000004    8        30\t75\tE0\t2E\t80\tFF\tFF\tFD\r\n      2423  0CF101A7   00000004    8        68\t00\t97\tCC\t00\t16\t39\t93\r\n      2422  1FFFFFFF   00000004    8        00\t00\tFF\tFF\tFF\tFF\tFF\tFF\r\n      2412  1FFFFFFF   00000004    8        00\t20\tFF\tFF\tFF\tFF\tFF\tFF\r\n      2403  0CF102A7   00000004    8        30\t75\tE0\t2E\t80\tFF\tFF\tFD\r\n      2403  0CF101A7   00000004    8        68\t00\t97\tCC\t00\t16\t39\t92\r\n      2444  0CF102A7   00000004    8        30\t75\tE0\t2E\t80\tFF\tFF\tFD\r\n      2443  0C3C4D4A   00000004    8        BE\tFF\tFF\t7F\t18\tFF\tFF\t50\r\n      2443  0CF101A7   00000004    8        68\t00\t97\tCC\t00\t16\t39\t94\r\n      2442  18F120F0   00000004    8        2B\t75\t60\tB1\tB0\t01\tFF\tFF\r\n      2441  18F11FF0   00000004    8        FF\t3F\t90\t68\t88\t1B\t10\t0C\r\n      2432  1FFFFFFF   00000004    8        00\t20\tFF\tFF\tFF\tFF\tFF\tFF\r\n      2423  0CF102A7   00000004    8        30\t75\tE0\t2E\t80\tFF\tFF\tFD\r\n      2423  0CF101A7   00000004    8        68\t00\t97\tCC\t00\t16\t39\t93\r\n      2422  1FFFFFFF   00000004    8        00\t00\tFF\tFF\tFF\tFF\tFF\tFF\r\n      2412  1FFFFFFF   00000004    8        00\t20\tFF\tFF\tFF\tFF\tFF\tFF\r\n      2403  0CF102A7   00000004    8        30\t75\tE0\t2E\t80\tFF\tFF\tFD\r\n      2444  0CF103A7   00000004    8        17\t1F\t08\t60\tB1\t1F\t08\t50\r\n      2444  0CF102A7   00000004    8        30\t75\tE0\t2E\t80\tFF\tFF\tFD\r\n      2443  0C3C4D4A   00000004    8        BE\tFF\tFF\t7F\t18\tFF\tFF\t50\r\n      2443  0CF101A7   00000004    8        68\t00\t97\tCC\t00\t16\t39\t94\r\n      2442  18F120F0   00000004    8        2B\t75\t60\tB1\tB0\t01\tFF\tFF\r\n      2441  18F11FF0   00000004    8        FF\t3F\t90\t68\t88\t1B\t10\t0C\r\n      2432  1FFFFFFF   00000004    8        00\t20\tFF\tFF\tFF\tFF\tFF\tFF\r\n      2423  0CF102A7   00000004    8        30\t75\tE0\t2E\t80\tFF\tFF\tFD\r\n      2423  0CF101A7   00000004    8        68\t00\t97\tCC\t00\t16\t39\t93\r\n      2422  1FFFFFFF   00000004    8        00\t00\tFF\tFF\tFF\tFF\tFF\tFF\r\n      2412  1FFFFFFF   00000004    8        00\t20\tFF\tFF\tFF\tFF\tFF\tFF\r\n      2445  0CF104A7   00000004    8        F0\t60\t22\tFC\tFF\tFF\tFF\t50\r\n      2444  0CF103A7   00000004    8        17\t1F\t08\t60\tB1\t1F\t08\t50\r\n      2444  0CF102A7   00000004    8        30\t75\tE0\t2E\t80\tFF\tFF\tFD\r\n      2443  0C3C4D4A   00000004    8        BE\tFF\tFF\t7F\t18\tFF\tFF\t50\r\n      2443  0CF101A7   00000004    8        68\t00\t97\tCC\t00\t16\t39\t94\r\n      2442  18F120F0   00000004    8        2B\t75\t60\tB1\tB0\t01\tFF\tFF\r\n      2441  18F11FF0   00000004    8        FF\t3F\t90\t68\t88\t1B\t10\t0C\r\n      2432  1FFFFFFF   00000004    8        00\t20\tFF\tFF\tFF\tFF\tFF\tFF\r\n      2423  0CF102A7   00000004    8        30\t75\tE0\t2E\t80\tFF\tFF\tFD\r\n      2423  0CF101A7   00000004    8        68\t00\t97\tCC\t00\t16\t39\t93\r\n      2422  1FFFFFFF   00000004    8        00\t00\tFF\tFF\tFF\tFF\tFF\tFF\r\n      2445  18F106A7   00000004    8        00\tF7\tFF\tFF\tFF\tFF\tFF\tA1\r\n      2445  0CF104A7   00000004    8        F0\t60\t22\tFC\tFF\tFF\tFF\t50\r\n      2444  0CF103A7   00000004    8        17\t1F\t08\t60\tB1\t1F\t08\t50\r\n      2444  0CF102A7   00000004    8        30\t75\tE0\t2E\t80\tFF\tFF\tFD\r\n      2443  0C3C4D4A   00000004    8        BE\tFF\tFF\t7F\t18\tFF\tFF\t50\r\n      2443  0CF101A7   00000004    8        68\t00\t97\tCC\t00\t16\t39\t94\r\n      2442  18F120F0   00000004    8        2B\t75\t60\tB1\tB0\t01\tFF\tFF\r\n      2441  18F11FF0   00000004    8        FF\t3F\t90\t68\t88\t1B\t10\t0C\r\n      2432  1FFFFFFF   00000004    8        00\t20\tFF\tFF\tFF\tFF\tFF\tFF\r\n      2423  0CF102A7   00000004    8        30\t75\tE0\t2E\t80\tFF\tFF\tFD\r\n      2423  0CF101A7   00000004    8        68\t00\t97\tCC\t00\t16\t39\t93\r\n      2446  18F121F0   00000004    8        09\t19\t00\t00\tFF\tFF\tB0\t01\r\n      2445  18F106A7   00000004    8        00\tF7\tFF\tFF\tFF\tFF\tFF\tA1\r\n      2445  0CF104A7   00000004    8        F0\t60\t22\tFC\tFF\tFF\tFF\t50\r\n      2444  0CF103A7   00000004    8        17\t1F\t08\t60\tB1\t1F\t08\t50\r\n      2444  0CF102A7   00000004    8        30\t75\tE0\t2E\t80\tFF\tFF\tFD\r\n      2443  0C3C4D4A   00000004    8        BE\tFF\tFF\t7F\t18\tFF\tFF\t50\r\n      2443  0CF101A7   00000004    8        68\t00\t97\tCC\t00\t16\t39\t94\r\n      2442  18F120F0   00000004    8        2B\t75\t60\tB1\tB0\t01\tFF\tFF\r\n      2441  18F11FF0   00000004    8        FF\t3F\t90\t68\t88\t1B\t10\t0C\r\n      2432  1FFFFFFF   00000004    8        00\t20\tFF\tFF\tFF\tFF\tFF\tFF\r\n      2423  0CF102A7   00000004    8        30\t75\tE0\t2E\t80\tFF\tFF\tFD\r\n      2447  1FFFFFFF   00000004    8        00\t20\tFF\tFF\tFF\tFF\tFF\tFF\r\n      2446  18F121F0   00000004    8        09\t19\t00\t00\tFF\tFF\tB0\t01\r\n      2445  18F106A7   00000004    8        00\tF7\tFF\tFF\tFF\tFF\tFF\tA1\r\n      2445  0CF104A7   00000004    8        F0\t60\t22\tFC\tFF\tFF\tFF\t50\r\n      2444  0CF103A7   00000004    8        17\t1F\t08\t60\tB1\t1F\t08\t50\r\n      2444  0CF102A7   00000004    8        30\t75\tE0\t2E\t80\tFF\tFF\tFD\r\n      2443  0C3C4D4A   00000004    8        BE\tFF\tFF\t7F\t18\tFF\tFF\t50\r\n      2443  0CF101A7   00000004    8        68\t00\t97\tCC\t00\t16\t39\t94\r\n      2442  18F120F0   00000004    8        2B\t75\t60\tB1\tB0\t01\tFF\tFF\r\n      2441  18F11FF0   00000004    8        FF\t3F\t90\t68\t88\t1B\t10\t0C\r\n      2432  1FFFFFFF   00000004    8        00\t20\tFF\tFF\tFF\tFF\tFF\tFF\r\n      2452  1FFFFFFF   00000004    8        00\t20\tFF\tFF\tFF\tFF\tFF\tFF\r\n      2447  1FFFFFFF   00000004    8        00\t20\tFF\tFF\tFF\tFF\tFF\tFF\r\n      2446  18F121F0   00000004    8        09\t19\t00\t00\tFF\tFF\tB0\t01\r\n
